vi "Load PID from File.vi"(8 "error in":errorcluster, 10 "Name":string, 11 "refnum in":T2) -> (0 "error out":errorcluster, 2 "PID":T1, 3 "refnum out":T2)   [LabVIEW 2016]
uses:
  <vilib>/Utility/config.llb/Config Data RefNum.ctl
  PID Settings.ctl
  <vilib>/Utility/config.llb/Read Key (Double).vi
  <vilib>/Utility/config.llb/NI_LVConfig.lvlib
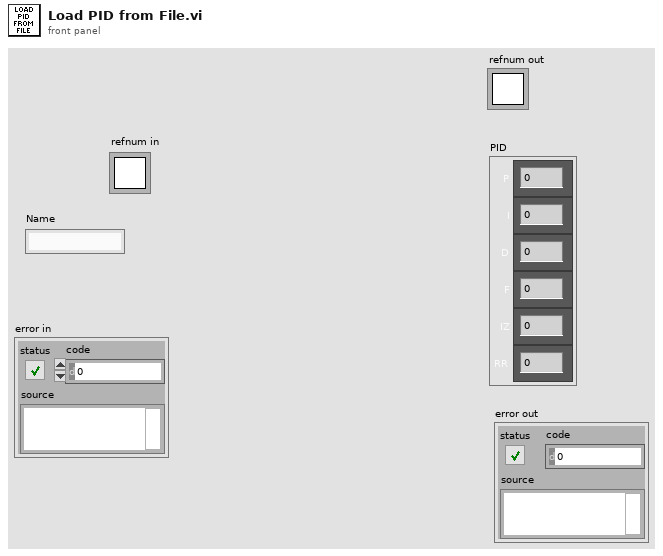
[diagram p1: front panel]
types:
  T1 = typedef "PID Settings.ctl" = cluster{"D":dbl, "F":dbl, "RR":dbl, "IZ":dbl, "P":dbl, "I":dbl}
  T2 = typedef "NI_LVConfig.lvlib/Config Data RefNum.ctl" = refnum<k1>
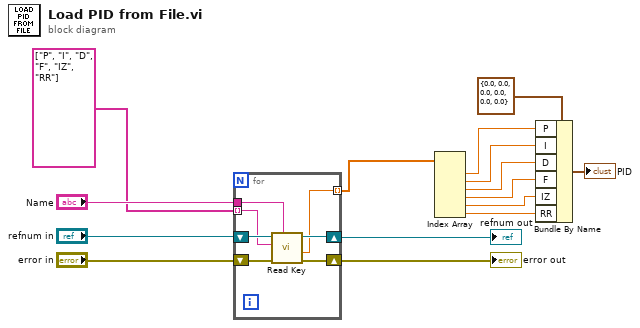
[diagram p0: block diagram]
diagram:
  n1 = for {
    tunnel: "Name" -> [w18]
    tunnel: string[] ["P", "I", "D", "F", "IZ", "RR"] -> [w19] mode=indexing
    shift-right: [w20] -> w10
    shift-left: "error in" -> [w21]
    shift-right: [w17] -> w11
    shift-left: "refnum in" -> [w22]
    tunnel: [w16] -> w1 mode=indexing
    n2 = call-poly <vilib>:"Read Key.vi"("section"=w18, "error in (no error)"=w21, "key"=w19, "refnum"=w22) -> ("error out"=w20:errorcluster, "value"=w16:dbl, "refnum out"=w17:T2)  [unwired: 4 in, 1 out]
  }
  "refnum out" <- w11
  "error out" <- w10
  n3 = Index Array(array=w1) -> (element #1=w8:dbl, element #2=w7:dbl, element #3=w6:dbl, element #4=w5:dbl, element #5=w4:dbl, element #6=w3:dbl)  [unwired: 6 in]
  n4 = Bundle By Name(cluster=T1 {"D"=0.0, "F"=0.0, "RR"=0.0, "IZ"=0.0, "P"=0.0, "I"=0.0} ("PID"), "P"=w8, "I"=w7, "D"=w6, "F"=w5, "IZ"=w4, "RR"=w3) -> (→"PID":T1)
